vi "AlliGator Special Graph Menu Actions.vi"(8 "Error In":errorcluster, 9 "Help?":bool, 10 "Animated Busy Icon":bool, 11 "XY Graph Event":T1) -> (0 "Error Out":errorcluster, 1 "Message":string, 3 "AlliGator Actions":T3[](array[typedef]))   [LabVIEW 2021, in "AlliGator Graphs.lvlib"]
doc: "Additional graph menu items developped for AlliGator."
uses:
  AlliGator Graphs.lvlib
  AlliGator Q Element.ctl
  AlliGator Q Event.ctl
  Graphs/XY Graph/XY Graph Event.ctl
  <vilib>/Utility/miscctls.llb/LVPoint32TypeDef.ctl
  Graphs/XY Graph/XY Graph Selected Plot Info.ctl
  Graphs/XY Graph/XY Graph Refnum.ctl
  AlliGator Decay Graph Process Plot Target.ctl
  Graphs/XY Graph/XY Graph Selected Plot Info+Flag.ctl
  AlliGator Variables List.ctl
  Graphs/XY Graph/XY Graph Add-Ons.lvlib
  AlliGator Action Engine.lvlib
  AlliGator Python Plugins.lvlib
  AlliGator Decay Processing.lvlib
  AlliGator Decay Analysis.lvlib
  AlliGator Globals, Variables & Constants.lvlib
panel:
  # "see the AlliGator License on the block diagram (Ctrl+E or Window:Show Block Diagram)"
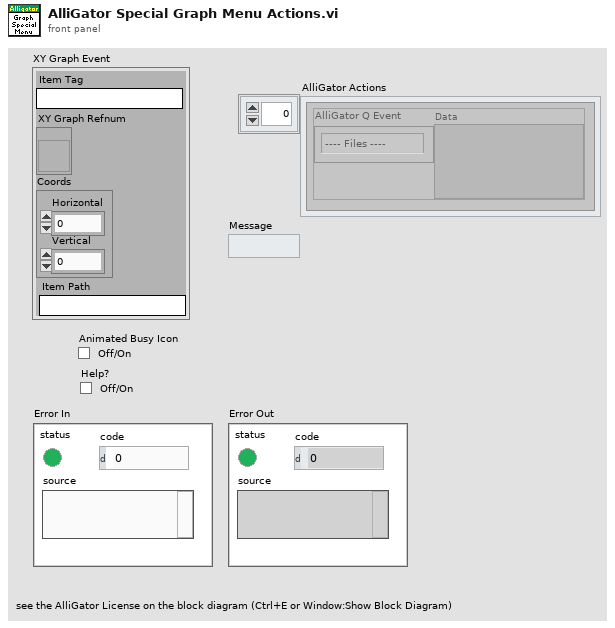
[diagram p1: front panel]
types:
  T1 = typedef "XY Graph Add-Ons.lvlib/XY Graph Event.ctl" = cluster{"Item Tag":string, "XY Graph Refnum":refnum<vi>, "Coords":T2, "Item Path":string}
  T2 = typedef "LVPoint32TypeDef.ctl" = cluster{"Horizontal":i32, "Vertical":i32}
  T3 = typedef "AlliGator Action Engine.lvlib/AlliGator Q Element.ctl" = cluster{"AlliGator Q Event":T4, "Data":variant}
  T4 = typedef "AlliGator Action Engine.lvlib/AlliGator Q Event.ctl" = enum16{"---- Files ----", "Files:Set Batch Export Files To Save", "Files:Set Dataset Loading & Pre-processing Options", "Files:Check #Frames in Dataset", "Files:Increment Frame Index", "Files:Open Mask Image", "Files:Open White Light Image", "Files:Open Single Dataset", "Files:New Folder of Folders Selected", "Files:Load File (all Types)_Scriptable", "Files:Move Flattened Series to Folders Series", "Files:Select Folder", "Files:Load FLI Dataset", "Files:Load Swiss SPAD 1 Dataset", "Files:Load Swiss SPAD 2 Dataset", "Files:Load .sdt FLI Dataset", "Files:Load .ptu FLI Dataset", "Files:Load .bin FLI Dataset", "Files:Load Single Gate Image Folder", "Files:Load I/m/phi Dataset (deprecated)", "Files:Load Single Image", "Files:Subtract Background File", "Files:Export FLI Dataset", "Files:Load HDF5 FLI Dataset", "Files:Set Destination File Path", "Files:Save Mask Image", "Files:Batch Conversion", "Files:New Folder Selected", "Files:Close FLI Dataset", "Files:Close FLI Dataset Series", "Files:Close White Light Image", "Files:Close Mask Image", "---- FLI Dataset ----", "FLI Dataset:Channel Arithmetic", "FLI Dataset:Export Average Lifetime Map as ASCII", "FLI Dataset:Export User-Defined Quantity Map as ASCII", "FLI Dataset:Python Function FLI Dataset Event", "FLI Dataset:ROI Analysis", "FLI Dataset:Tilted Logistic Square Gated IRF Characteristics Map", "FLI Dataset:Logistic Square Gated IRF Characteristics Map", "FLI Dataset:Square Gated IRF Characteristics Map", "FLI Dataset:Multi-ROI Single-Pixel Phasor Analysis", "FLI Dataset:Multi-ROI Single-Pixel NLSF Analysis", "FLI Dataset:All ROIs IRF Extraction", "FLI Dataset:All ROIs Decay Fit Non-Interactive (Fast + Individual IRF)", "FLI Dataset:All ROIs Phasor Analysis", "FLI Dataset:All ROIs Decay Fit", "FLI Dataset:Fluorescence Decay Statistics", "FLI Dataset:Update Decay Statistics Graph", "FLI Dataset:Get Decay from ROI", "FLI Dataset:All ROIs Average Lifetimes", "---- FLI Dataset Series ----", "FLI Dataset Series:Sum All Datasets in Series", "FLI Dataset Series:Add Dataset to Accumulated Dataset", "FLI Dataset Series:Display Accumulated Dataset", "FLI Dataset Series:Clear Dataset Series Sum", "FLI Dataset Series:Time-Series Analysis (NLSF)", "FLI Dataset Series:Time-Series Analysis (Phasor)", "---- Image ----", "Image:Update Image Profile Plots", "Image:Image Histogram Cursor Move", "Image:Image Histogram", "Image:Image Contrast", "Image:Set Image Histogram Cursor Move Flag", "Image:Clear Image Overlay", "Image:Use ROI as Search Area", "Image:Set ROI Diameter", "Image:Save Image Data as TIFF", "Image:Save Displayed Image with Overlay", "Image:Save Image Overlay Only", "Image:Save Image as Hot Pixel Mask", "Image:Change Source Image Color Palette", "Image:Copy Image to Clipboard", "Image:Source Image ROI Selection", "Image:Delete All ROIs", "Image:Delete All Unselected ROIs", "Image:Delete ROI", "Image:Merge All ROIs", "Image:Store ROI", "Image:Source Image ROI Storage", "Image:Export ROI Description to Notebook", "Image:Save ROI", "Image:Load ROI", "Image:Paste ROI Definition", "Image:Clear ROI", "Image:Identify ROIs in Mask Image", "Image:Create Complementary ROI", "Image:Create Contour ROI", "Image:Create ROI(s) from Pixels with Peak above Min_Scriptable", "Image:Create ROI(s) from Pixels with Intensity above Min_Scriptable", "Image:Compute ROI Statistics", "Image:Delete ROI(s) based on ROI Statistics", "Image:Create ROI Grid", "Image:ROI to Individual Pixel ROIs", "Image:Python Function Source Image Event", "Image:Show Phasor Calibration Map ROI Centers", "Image:Convert ROI to Mask Image", "Image:Mouse Move", "Image:Mouse Up", "Image:Set Source Image Mouse Move Flag", "Image:Add Scale Bar Overlay", "Image:Delete Existing ROIs Option", "---- Decay ----", "Decay:Clear IRF/Reference Plot", "Decay:Clear Local IRFs", "Decay:Add Decay to Graph", "Decay:Smoothen Plot", "Decay:Smoothen Plot Tail", "Decay:Average Selected Plots", "Decay:Extract IRF", "Decay:Optimal IRF Extraction", "Decay:Threshold IRF", "Decay:Fit to Model IRF", "Decay:Fit IRF to Square Gate", "Decay:Fit IRF to Logistic Square Gate", "Decay:Fit IRF to Tilted Logistic Square Gate", "Decay:Create Bounding Cursors Set", "Decay:Export Bounding Cursors Definition to Notebook", "Decay:Denoise Plot", "Decay:Compute Cumulative Function", "Decay:Use as Reference Decay", "Decay:Show Reference Decay/IRF", "Decay:Extrapolate Decay", "Decay:Create Head & Tail Bounding Cursors", "Decay:Store Cursor-defined Head & Tail Fractions", "Decay:Rebin Plot", "Decay:1-Normalize Decay", "Decay:[0-1]-Normalize Plot", "Decay:Straighten Decay", "Decay:Shift Decay", "Decay:Fold Decay", "Decay:Fit Decay", "Decay:Global Fit of Selected Decays", "Decay:Post Global Fit Script", "Decay:Add Global Fit Parameters to Graph", "Decay:Add Decay Parameter(s) to Plot (Graph)", "Decay:Export Decay to Phasor Graph", "Decay:Plot Decay Shifts", "Decay:Compute Average Lifetime", "Decay:Plot Convolution", "Decay:Graph Tip Strip Update", "---- Decay Statistics ----", "Decay Statistics:Tip Strip Update", "---- Intensity Time Trace ----", "Intensity Time Trace:Use File Timestamp", "Intensity Time Trace:Load Intensity Corrections File", "Intensity Time Trace:Clear Intensity Corrections File", "Intensity Time Trace:Tip Strip Update", "---- Phasor Plot ----", "Phasor Plot:Build Phasor Plot", "Phasor Plot:Change Phasor Plot Color Palette", "Phasor Plot:Adjust Phasor Plot Display Range", "Phasor Plot:Highlight Image ROI in Phasor Plot", "Phasor Plot:Save Phasor Plot Image with Overlay", "Phasor Plot:Export Complex Phasor Map", "Phasor Plot:Export Phasor Ratio Map", "Phasor Plot:Export Average Lifetime Map", "Phasor Plot:Compute Phase Lifetime Histogram", "Phasor Plot:Compute Phasor Ratio Histogram", "Phasor Plot:Compute Phase Lifetime vs Intensity Scatter Plot", "Phasor Plot:Weber 2-Component Decomposition", "Phasor Plot:Update Phasor Color Map Vertices", "Phasor Plot:Clear Phasor Overlay", "Phasor Plot:Use Segment Extremities as References", "Phasor Plot:Use UC/Segment Intersections as References", "Phasor Plot:Use UC/Principal Axis Intersections as References", "Phasor Plot:Use UC/Linear Fit Intersections as References", "Phasor Plot:Update Phasor Plot Reference", "Phasor Plot:Show Local Phasor Info in Phasor Plot", "Phasor Plot:Update Phasor Plot State", "Phasor Plot:Phasor Plot ROI Storage", "Phasor Plot:Phasor Plot ROI Selection", "Phasor Plot:Python Function Phasor Plot Event", "Phasor Plot:Overlay Phasor ROI, Ratio or Map in Source Image", "Phasor Plot:Phasor at Image Pixel", "Phasor Plot:Mouse Move", "Phasor Plot:Mouse Up", "Phasor Plot:Display Range Mouse Move", "Phasor Plot:Set Mouse Move Flag", "---- Phasor Graph ----", "Phasor Graph:Calibrated Phasor Map Series", "Phasor Graph:Whole Image Phasor Scatter Plot (Todo)", "Phasor Graph:Get Phasor Value", "Phasor Graph:Create New Phasor Plot Dialog", "Phasor Graph:Update Last Phasor Value", "Phasor Graph:Update Phasor (m, phi)", "Phasor Graph:Remove Single Phasor from Plot", "Phasor Graph:Add Single Phasor to Plot", "Phasor Graph:Remove Phasor Plot", "Phasor Graph:Remove Selected Phasor Plots", "Phasor Graph:Clear Phasor Data", "Phasor Graph:Clear Phasor Graph", "Phasor Graph:Cursor Move", "Phasor Graph:Draw Cursor Connecting Line", "Phasor Graph:Clear Cursor Connecting Line", "Phasor Graph:Find UC Intersection", "Phasor Graph:Use UC/Cursor-Defined Line Intersections", "Phasor Graph:Use Selected Plots Fitted Line/UC Intersections", "Phasor Graph:Use Selected Plots Principal Axis/UC Intersections", "Phasor Graph:Show Single Phasor", "Phasor Graph:Save Single Phasor Plot", "Phasor Graph:Save All Phasor Plots", "Phasor Graph:Load Phasor Plot(s)", "Phasor Graph:Phasor Multiplication", "Phasor Graph:Compute Average Phasor", "Phasor Graph:Compute Multiple Average Phasors (Selected Plots)", "Phasor Graph:Export Single Phasor Plot Phase Lifetimes", "Phasor Graph:Phase Lifetime Trajectory", "Phasor Graph:Phase Lifetime vs Intensity Scatter Plot (deprecated)", "Phasor Graph:Parameter 2 vs Parameter 1 Scatter Plot", "Phasor Graph:Use Cursor n Location", "Phasor Graph:Set Reference n to Current Phase Lifetime Value", "Phasor Graph:Set Reference n to Lifetime Value", "Phasor Graph:Set Cursor n Location", "Phasor Graph:Save Phasor Graph Image", "Phasor Graph:Update SEPL Plot", "Phasor Graph:Export Single Phasor Plot Data", "Phasor Graph:Export Selected Phasor Plots Data", "Phasor Graph:Python Function Phasor Graph Event", "Phasor Graph:Tip Strip Update", "---- Calibration ----", "Calibration:Set Calibration Type", "Calibration:Load/Save Phasor Calibration", "Calibration:Load/Save Phasor Calibration Series", "Calibration:Load/Save Phasor Calibration Map", "Calibration:Use as Calibration", "Calibration:Compute Optimal Calibration from Phasor References", "Calibration:Clear Phasor Calibration", "Calibration:Use as Calibration Series", "Calibration:Use as Calibration Map", "Calibration:Clear Calibration Series", "Calibration:Clear Calibration Map", "Calibration:Apply Phasor Calibration", "Calibration:Update Single Plot Calibration", "Calibration:Update Multiple Plots Calibration", "Calibration:Clear Single Plot Calibration", "Calibration:Clear All Plots Calibrations", "Calibration:Clear Plot(s) Calibration(s)?", "Calibration:Phasor Calibration Maps (# Gates Series)", "---- Phasor Ratio ----", "Phasor Ratio:Clear Reference n", "Phasor Ratio:Toggle Selected Plot(s)  Lock to Reference 1", "Phasor Ratio:Use as Reference n", "Phasor Ratio:Send Reference n to Notebook", "Phasor Ratio:Toggle Selected Plot(s)  Lock to Reference 2", "Phasor Ratio:Compute Phasor Ratio at Mouse Location", "Phasor Ratio:Compute Phasor Plot's Average Phasor Ratio", "Phasor Ratio:Compute Time-Series Phasor Ratios", "Phasor Ratio:Fit Line to Phasor Ratio Plot", "Phasor Ratio:Save References", "Phasor Ratio:Load References", "Phasor Ratio:Update Phasor Reference 1", "Phasor Ratio:Update Phasor Reference 2", "Phasor Ratio:Move Cursor n to Reference n", "Phasor Ratio:Use as Phasor Reference 1 Lifetime", "Phasor Ratio:Use as Phasor Reference 2 Lifetime", "Phasor Ratio:Export Phasor Ratio Map as ASCII", "Phasor Ratio:Tip Strip Update", "---- Lifetime & Other Parameters Graph ----", "Lifetime:Tip Strip Update", "---- Decay Fit Parameter Map ----", "Decay Fit Parameter Map:Export ROI NLSF Data as ASCII", "Decay Fit Parameter Map:Set Decay Fit  Parameter Map Selection", "Decay Fit Parameter Map:Build Decay Fit Parameter Map", "Decay Fit Parameter Map:Change Decay Fit Parameter Map Color Palette", "Decay Fit Parameter Map:Export Decay Fit Parameter Map Data as ASCII", "Decay Fit Parameter Map:Export All Decay Fit Parameter Maps Data as ASCII", "Decay Fit Parameter Map:Send Map Data to Lifetime Graph", "Decay Fit Parameter Map:Save Decay Fit Parameter Map Image", "Decay Fit Parameter Map:Save-Load IRFs & Fit Data", "Decay Fit Parameter Map:Update Local Decay Plots", "Decay Fit Parameter Map:Python Function Decay Fit Parameters Map Event", "Decay Fit Parameter Map:Overlay Decay Fit Parameter Map in Source Image", "Decay Fit Parameter Map:Plot Map Data vs Intensity", "Decay Fit Parameter Map:Mouse Up", "Decay Fit Parameter Map:Display Range Mouse Move", "---- Generic Graph ----", "Generic Graph:Generic XY Graph Event", "Generic Graph:Python Function XY Graph Event", "Generic Graph:New Plot", "Generic Graph:Save Plot", "Generic Graph:XY Plot Histogram", "Generic Graph:Set XY Graph Plot Name", "Generic Graph:Set Last Cursor Style", "Generic Graph:Tip Strip Update", "---- GUI ----", "GUI:Start Script", "GUI:Type of Displayed Image Changed", "GUI:Gate Image Slide Changed", "GUI:Show Busy Icon", "GUI:Show Busy Icon & Abort Button", "GUI:Hide Busy Icon", "GUI:Hide Busy Icon & Abort Button", "GUI:Abort", "GUI:End Script", "GUI:Start Timing", "GUI:End Timing", "GUI:Set State Indicator", "GUI:Send Parameters JSON Strings to Clipboard", "GUI:Set Gate Step", "GUI:Idle", "GUI:Initialization", "GUI:Quit", "GUI:Increment Dataset Index", "GUI:Set Dataset Index to -1", "GUI:Time Series Slider Moved", "GUI:Time Series Slider Changed", "GUI:Toggle Playback or Loop", "GUI:Playback Script", "GUI:Set Phasor Frequency", "GUI:Open Window", "DEBUG"}
  T5 = typedef "XY Graph Add-Ons.lvlib/XY Graph Selected Plot Info.ctl" = cluster{"Multiplot XY Graph":T6, "Mouse Coordinates":T2, "Plot Index":i32}
  T6 = typedef "XY Graph Add-Ons.lvlib/XY Graph Refnum.ctl" = refnum<vi>
  T7 = typedef "AlliGator Decay Analysis.lvlib/AlliGator Decay Graph Process Plot Target.ctl" = enum16{"Single Plot", "Selected Plots", "All Plots"}
  T8 = typedef "XY Graph Add-Ons.lvlib/XY Graph Selected Plot Info+Flag.ctl" = cluster{"Multiplot XY Graph":T6, "Mouse Coordinates":T2, "Plot Index":i32, "Flag":bool}
  T9 = typedef "AlliGator Globals, Variables & Constants.lvlib/AlliGator Variables List.ctl" = enum16{"---- GUI ----", "Initialization Status", "State Indicators Refnum", "Original AlliGator Menu Items", "Current Action Loop State", "Script in progress", "Playback", "Loop Playback", "Search ROI Used", "Search ROI", "Decay Graph Max Legend Size", "Intensity Graph Max Legend Size", "Decay Statistics Graph Max Legend Size", "Phasor Graph Max Legend Size", "Phasor Ratio Graph Max Legend Size", "Lifetime Graph Max Legend Size", "---- Files ----", "Export Dataset Frames as Individual Files", "Show Batch Export Help Balloons", "Frames in Dataset", "ptu File Frame Start Indices", "Current Frame in Dataset", "Current Frame Timestamp", "------ Python Plugins ------", "Python Plugins Information", "Python Session", "Valid Python Session?", "---- Source Image ----", "Dataset Loaded", "Dataset Metadata", "Dataset Channel", "Dataset Data Description", "Background Dataset Metadata", "Background Dataset Channel", "Background Dataset Data Description", "Background File Subtraction", "Background File Path", "Background File Pile-up Correction", "Background File Pixel Well Capacity", "Background File Scaling Factor", "Source Image ROIs", "Current Source Image ROI", "Source Image ROI Event Refnum", "X_Source Image Display Range", "X_Source Image Palette Information", "Source Image Palette List", "Source Image Scale", "Current Dataset Load Settings", "Source Image:ROI Overlay Color", "---- Image Profile Window ----", "Image Profile:Overlay ROI in Source Image", "Image Profile Window Event Refnum", "Image Profile:IntensityType", "Image Profile:Intensity Average Type", "Image Profile:Intensity-weighted SDV", "Image Profile:Box Profile Type", "Image Profile Window Open", "Image Profile:Plotted Fit Parameter", "X_Type of Displayed Image", "X_Time Gate Slider", "Dataset Path", "Source Image Overlay to Erase", "Is Displayed Image Accumulated", "White Light Image Modified", "Mask Image Modified", "Macrotime Gate Separation", "------ Phasor Graph -------", "Phasor Graph:Show Line", "---- Phasor Plot ---", "Phasor Plot Parameters Changed", "FLI Dataset Modified since last Phasor Plot Calculation", "Phasor Harmonics Data", "Selected Phasor Harmonics", "Phasor Harmonic Manager Event Refnum", "Phasor Plot ROIs", "Current Phasor Plot ROI", "Phasor Plot ROI Event Refnum", "Phasor Plot Image Reference Points", "Phasor Plot Computed", "Phasor Plot Palette Information", "Phasor Plot Palette List", "Phasor Ratio Palette Information", "Phasor Ratio Palette List", "Phasor Image Scale", "Phasor Plot Image Overlay to Erase", "Phasor Plot Image Elements to Update", "Current Phasor Plot Calculation Parameters", "Current Phasor Calibration Options", "Reset Cumulated Phasor Plot", "Phasor Ratio Reference 1", "Phasor Ratio Lifetime Reference 1", "Phasor Ratio Reference 1 Frequency", "Phasor Ratio Reference 2", "Phasor Ratio Lifetime Reference 2", "Phasor Ratio Reference 2 Frequency", "---- Decay Analysis ----", "Number of Selected Decays to Fit", "LS Fit Results", "LAR Fit Results", "BS Fit Results", "Last Decay Max - Min", "Best Fit Parameters", "Best Fit Parameter Names", "Actual Size X", "Actual Size Y", "Binning X", "Binning Y", "Actual # Gates", "Dataset Number", "Gates to...", "Gates Skipped", "Gates to keep", "Gate Step", "Gate Separation", "Reversed Gates", "Pile-up Correction", "Pixel Well Capacity", "Background Subtracted", "Background Subtraction Method", "Background Definition Range", "Background File (deprecated)", "Number of Dataset Accumulated", "Array of Accumulated Dataset Paths", "Do Averaged Datasets", "Destination File Path", "Process Plot Target", "Use 1/D as Phasor Frequency", "---- Decay Fit Parameter Map -----", "Decay Fit Parameter Map Palette Information", "Decay Fit Parameter Map Palette List", "Local Decay Graph Window Event Refnum", "------- Local Decay Window ---------", "Use normalized IRF for convolution", "----- Miscellaneous ----", "Skippable Dialog Windows Status"}
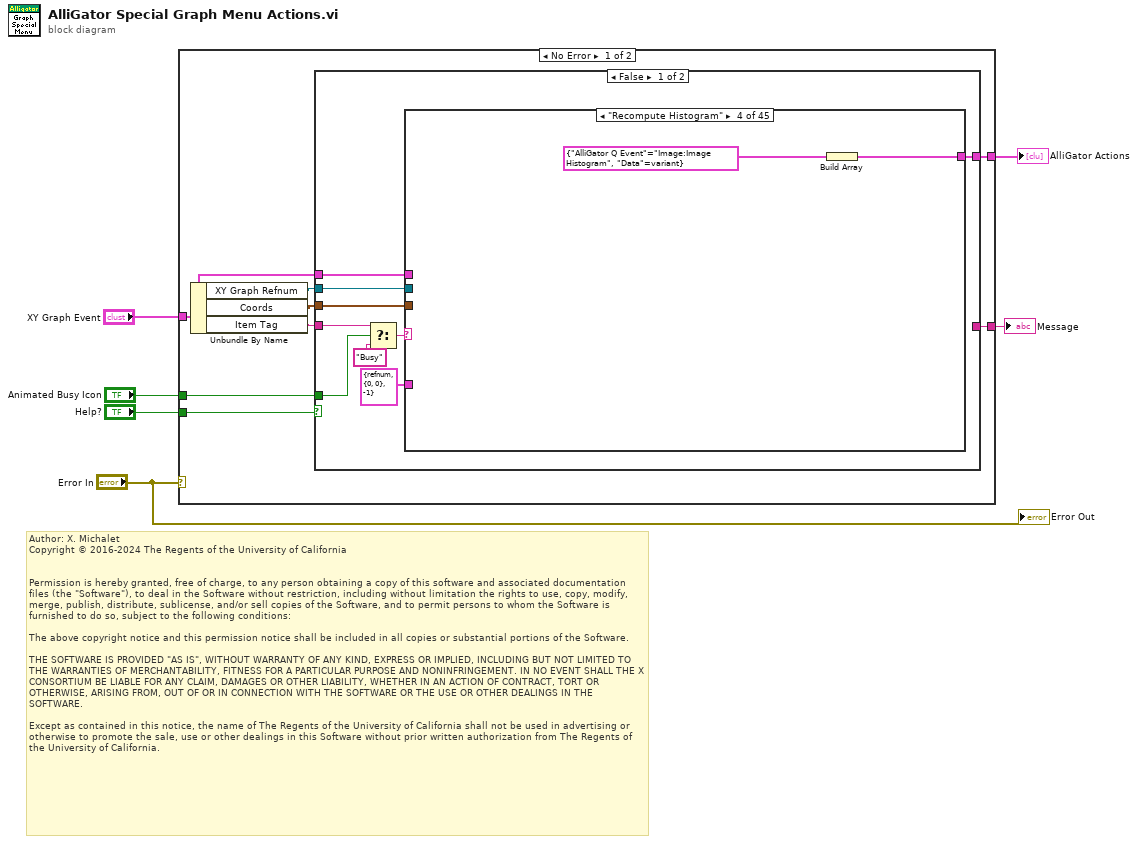
[diagram p0: block diagram]
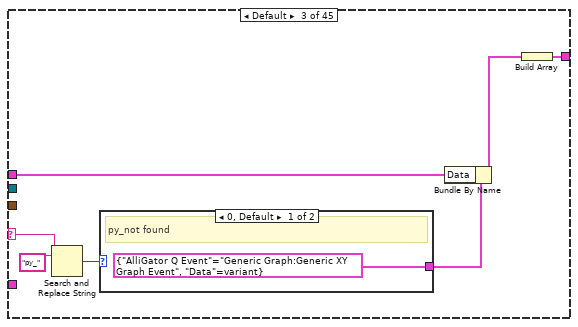
[diagram p4: hidden frame]
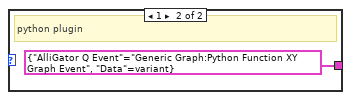
[diagram p5: hidden frame]
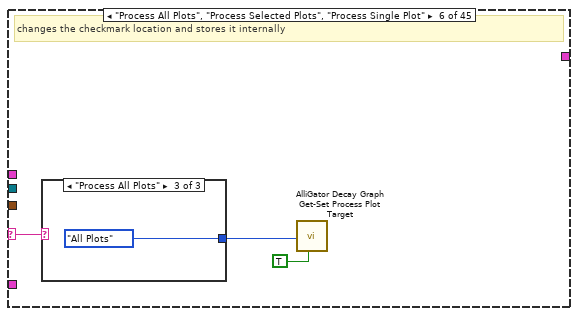
[diagram p7: hidden frame]
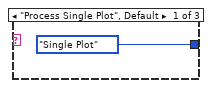
[diagram p8: hidden frame]
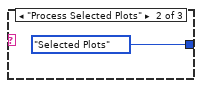
[diagram p9: hidden frame]
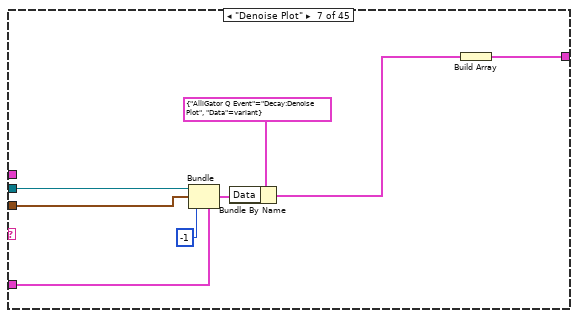
[diagram p10: hidden frame]
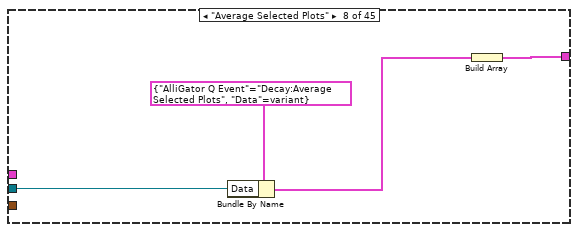
[diagram p11: hidden frame]
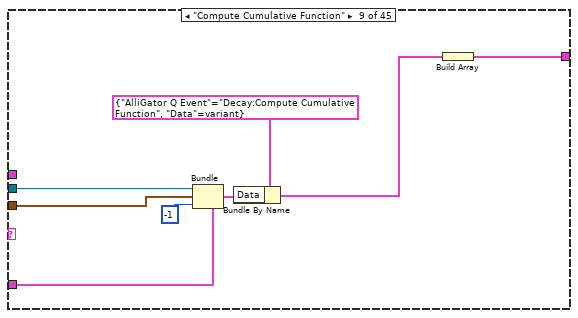
[diagram p12: hidden frame]
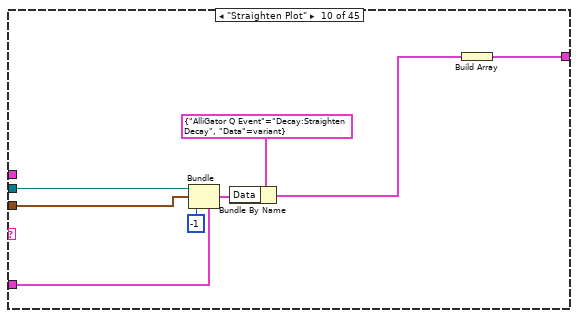
[diagram p13: hidden frame]
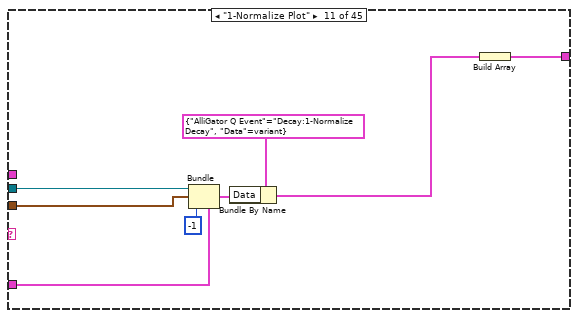
[diagram p14: hidden frame]
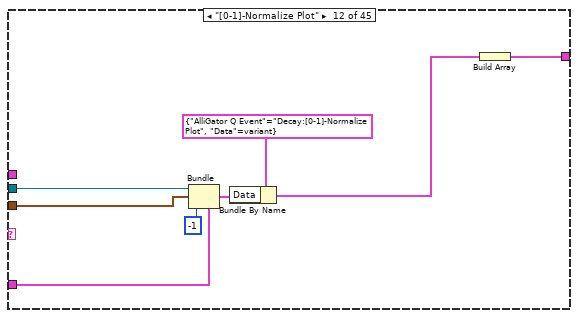
[diagram p15: hidden frame]
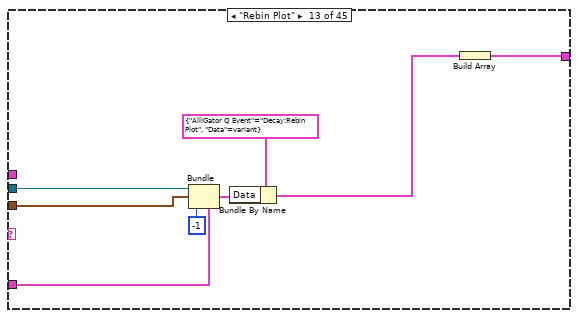
[diagram p16: hidden frame]
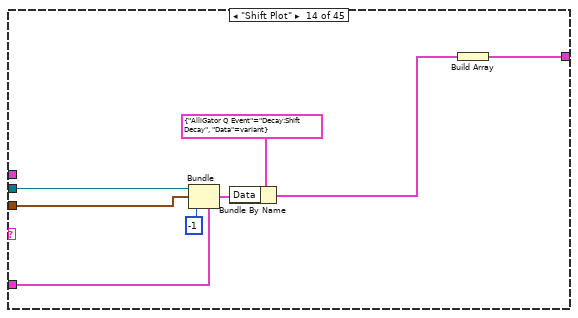
[diagram p17: hidden frame]
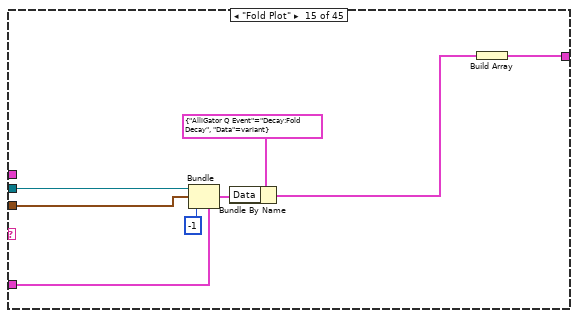
[diagram p18: hidden frame]
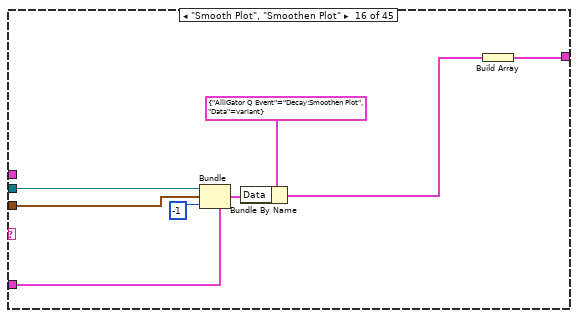
[diagram p19: hidden frame]
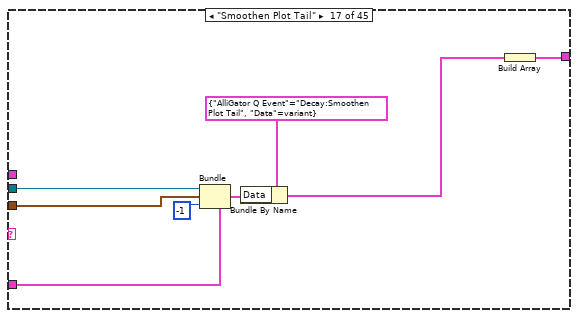
[diagram p20: hidden frame]
diagram:
  # "Author: X. Michalet\nCopyright © 2016-2024 The Regents of the University of California\n \n\nPermission is hereby granted, free of charge, to any person obtaining a copy of this software and associated documentation files (the \"Software\"), to deal in the Software without restriction, including without limitation the rights to use, copy, modify, merge, publish, distribute, sublicense, and/or sell copies of the Software, and to permit persons to whom the Software is furnished to do so, subject to the following conditions:\n\nThe above copyright notice and this permission notice shall be included in all copies or substantial portions of the Software.\n\nTHE SOFTWARE IS PROVIDED \"AS IS\", WITHOUT WARRANTY OF ANY KIND, EXPRESS OR IMPLIED, INCLUDING BUT NOT LIMITED TO THE WARRANTIES OF MERCHANTABILITY, FITNESS FOR A PARTICULAR PURPOSE AND NONINFRINGEMENT. IN NO EVENT SHALL THE X CONSORTIUM BE LIABLE FOR ANY CLAIM, DAMAGES OR OTHER LIABILITY, WHETHER IN AN ACTION OF CONTRACT, TORT OR OTHERWISE, ARISING FROM, OUT OF OR IN CONNECTION WITH THE SOFTWARE OR THE USE OR OTHER DEALINGS IN THE SOFTWARE.\n\nExcept as contained in this notice, the name of The Regents of the University of California shall not be used in advertising or otherwise to promote the sale, use or other dealings in this Software without prior written authorization from The Regents of the University of California."
  n1 = case shown="No Error" "Error In" {
    tunnel: [w14 _] -> w6
    tunnel: "Help?" -> [w13 _]
    tunnel: "Animated Busy Icon" -> [w12 _]
    tunnel: "XY Graph Event" -> [w8 _]
    tunnel: [w7 _] -> w1
    frame No Error {
      n2 = Unbundle By Name(w8) -> ("XY Graph Refnum"=w11:refnum<vi>, "Coords"=w10:T2, "Item Tag"=w9:string)
      n3 = case shown="False" w13 {
        tunnel: w12 -> [w23 _]
        tunnel: w9 -> [w21 w279]
        tunnel: w11 -> [w20 w281]
        tunnel: w10 -> [w19 _]
        tunnel: [w17 _] -> w14
        tunnel: w8 -> [w15 _]
        tunnel: [_ w278] -> w7
        frame False {
          n4 = Select(t=w21, s=w23, f="Busy" ("t")) -> (s? t:f=w22:string)
          n5 = case shown="\"Recompute Histogram\"" w22 {
            selector: w22 -> [_ _ w24 _ _ w37 _ _ _ _ _ _ _ _ _ _ _ _ _ _ _ _ _ _ _ _ _ _ _ _ _ _ _ _ _ _ _ _ _ _ _ _ _ _ _]
            tunnel: w20 -> [_ _ _ _ _ _ w46 w50 w58 w66 w74 w82 w90 w98 w106 w114 w122 w130 _ w140 w148 _ w156 _ w164 w172 w180 w188 w196 w202 w216 w224 _ _ _ w236 _ _ _ _ w251 _ _ w261 w272]
            tunnel: w19 -> [_ _ _ _ _ _ w44 _ w56 w64 w72 w80 w88 w96 w104 w112 w120 w128 _ w139 w147 _ w155 _ w162 w170 w178 w186 w194 w201 w214 w222 _ _ _ w234 _ _ _ _ w249 _ _ w260 w271]
            tunnel: T5 {"Multiplot XY Graph"=refnum, "Mouse Coordinates"={"Horizontal"=0, "Vertical"=0}, "Plot Index"=-1} ("Selected Plot Info") -> [_ _ _ _ _ _ w42 _ w54 w62 w70 w78 w86 w94 w102 w110 w118 w126 _ w135 w143 _ w151 _ w160 w168 w176 w184 w192 w200 w212 w220 _ _ _ w232 _ _ _ _ _ _ _ w262 w273]
            tunnel: [_ _ w26 w33 _ _ w41 w49 w53 w61 w69 w77 w85 w93 w101 w109 w117 w125 w133 w136 w144 _ w152 _ w159 w167 w175 w183 w191 w199 w211 w219 w227 w229 _ w231 w239 w242 w244 _ w245 w254 _ w259 w270] -> w17
            tunnel: w15 -> [_ _ w25 _ _ _ _ _ _ _ _ _ _ _ _ _ _ _ _ _ _ _ _ _ _ _ _ _ _ _ _ _ _ _ _ _ _ _ _ _ _ _ _ _ _]
            frame "-" {
            }
            frame "Busy" {
            }
            frame Default {
              n6 = Search and Replace String(input string=w24, search string="py_") -> (number of replacements=w27:i32)  [unwired: 6 in, 3 out]
              n7 = case shown="0, Default" w27 {
                tunnel: [T3 {"AlliGator Q Event"=enum."Generic Graph:Generic XY Graph Event", "Data"=variant} ("element") T3 {"AlliGator Q Event"=enum."Generic Graph:Python Function XY Graph Event", "Data"=variant} ("element")] -> w29
                frame 0, Default {
                  # "py_not found"
                }
                frame 1 {
                  # "python plugin"
                }
              }
              n8 = Bundle By Name(cluster=w29, "Data"=w25) -> (w28:T3)
              n9 = Build Array(w28) -> (w26:T3[])
            }
            frame "Recompute Histogram" {
              n10 = Build Array(T3 {"AlliGator Q Event"=enum."Image:Image Histogram", "Data"=variant} ("element")) -> (w33:T3[])
            }
            frame "---------------------" {
            }
            frame "Process All Plots", "Process Selected Plots", "Process Single Plot" {
              # "changes the checkmark location and stores it internally"
              n11 = case shown="\"Process All Plots\"" w37 {
                tunnel: [AlliGator_Decay_Graph_Process_Plot_Target."Single Plot" ("Process Plot Target") AlliGator_Decay_Graph_Process_Plot_Target."Selected Plots" ("Process Plot Target") AlliGator_Decay_Graph_Process_Plot_Target."All Plots" ("Process Plot Target")] -> w36
                frame "Process Single Plot", Default {
                }
                frame "Process Selected Plots" {
                }
                frame "Process All Plots" {
                }
              }
              n12 = call "AlliGator Decay Graph Get-Set Process Plot Target.vi"("Get (F)/Set"=TRUE, "Plot(s) to Process in"=w36) -> ()  [unwired: 7 in, 3 out]
            }
            frame "Denoise Plot" {
              n13 = Bundle(cluster=w42, "Multiplot XY Graph"=w46, "Mouse Coordinates"=w44, "Plot Index"=-1) -> (w45:T5)
              n14 = Bundle By Name(cluster=T3 {"AlliGator Q Event"=enum."Decay:Denoise Plot", "Data"=variant} ("element"), "Data"=w45) -> (w47:T3)
              n15 = Build Array(w47) -> (w41:T3[])
            }
            frame "Average Selected Plots" {
              n16 = Bundle By Name(cluster=T3 {"AlliGator Q Event"=enum."Decay:Average Selected Plots", "Data"=variant} ("element"), "Data"=w50) -> (w51:T3)
              n17 = Build Array(w51) -> (w49:T3[])
            }
            frame "Compute Cumulative Function" {
              n18 = Bundle(cluster=w54, "Multiplot XY Graph"=w58, "Mouse Coordinates"=w56, "Plot Index"=-1) -> (w57:T5)
              n19 = Bundle By Name(cluster=T3 {"AlliGator Q Event"=enum."Decay:Compute Cumulative Function", "Data"=variant} ("element"), "Data"=w57) -> (w59:T3)
              n20 = Build Array(w59) -> (w53:T3[])
            }
            frame "Straighten Plot" {
              n21 = Bundle(cluster=w62, "Multiplot XY Graph"=w66, "Mouse Coordinates"=w64, "Plot Index"=-1) -> (w65:T5)
              n22 = Bundle By Name(cluster=T3 {"AlliGator Q Event"=enum."Decay:Straighten Decay", "Data"=variant} ("element"), "Data"=w65) -> (w67:T3)
              n23 = Build Array(w67) -> (w61:T3[])
            }
            frame "1-Normalize Plot" {
              n24 = Bundle(cluster=w70, "Multiplot XY Graph"=w74, "Mouse Coordinates"=w72, "Plot Index"=-1) -> (w73:T5)
              n25 = Bundle By Name(cluster=T3 {"AlliGator Q Event"=enum."Decay:1-Normalize Decay", "Data"=variant} ("element"), "Data"=w73) -> (w75:T3)
              n26 = Build Array(w75) -> (w69:T3[])
            }
            frame "[0-1]-Normalize Plot" {
              n27 = Bundle(cluster=w78, "Multiplot XY Graph"=w82, "Mouse Coordinates"=w80, "Plot Index"=-1) -> (w81:T5)
              n28 = Bundle By Name(cluster=T3 {"AlliGator Q Event"=enum."Decay:[0-1]-Normalize Plot", "Data"=variant} ("element"), "Data"=w81) -> (w83:T3)
              n29 = Build Array(w83) -> (w77:T3[])
            }
            frame "Rebin Plot" {
              n30 = Bundle(cluster=w86, "Multiplot XY Graph"=w90, "Mouse Coordinates"=w88, "Plot Index"=-1) -> (w89:T5)
              n31 = Bundle By Name(cluster=T3 {"AlliGator Q Event"=enum."Decay:Rebin Plot", "Data"=variant} ("element"), "Data"=w89) -> (w91:T3)
              n32 = Build Array(w91) -> (w85:T3[])
            }
            frame "Shift Plot" {
              n33 = Bundle(cluster=w94, "Multiplot XY Graph"=w98, "Mouse Coordinates"=w96, "Plot Index"=-1) -> (w97:T5)
              n34 = Bundle By Name(cluster=T3 {"AlliGator Q Event"=enum."Decay:Shift Decay", "Data"=variant} ("element"), "Data"=w97) -> (w99:T3)
              n35 = Build Array(w99) -> (w93:T3[])
            }
            frame "Fold Plot" {
              n36 = Bundle(cluster=w102, "Multiplot XY Graph"=w106, "Mouse Coordinates"=w104, "Plot Index"=-1) -> (w105:T5)
              n37 = Bundle By Name(cluster=T3 {"AlliGator Q Event"=enum."Decay:Fold Decay", "Data"=variant} ("element"), "Data"=w105) -> (w107:T3)
              n38 = Build Array(w107) -> (w101:T3[])
            }
            frame "Smooth Plot", "Smoothen Plot" {
              n39 = Bundle(cluster=w110, "Multiplot XY Graph"=w114, "Mouse Coordinates"=w112, "Plot Index"=-1) -> (w113:T5)
              n40 = Bundle By Name(cluster=T3 {"AlliGator Q Event"=enum."Decay:Smoothen Plot", "Data"=variant} ("element"), "Data"=w113) -> (w115:T3)
              n41 = Build Array(w115) -> (w109:T3[])
            }
            frame "Smoothen Plot Tail" {
              n42 = Bundle(cluster=w118, "Multiplot XY Graph"=w122, "Mouse Coordinates"=w120, "Plot Index"=-1) -> (w121:T5)
              n43 = Bundle By Name(cluster=T3 {"AlliGator Q Event"=enum."Decay:Smoothen Plot Tail", "Data"=variant} ("element"), "Data"=w121) -> (w123:T3)
              n44 = Build Array(w123) -> (w117:T3[])
            }
            frame "Extrapolate Plot" {
              n45 = Bundle(cluster=w126, "Multiplot XY Graph"=w130, "Mouse Coordinates"=w128, "Plot Index"=-1) -> (w129:T5)
              n46 = Bundle By Name(cluster=T3 {"AlliGator Q Event"=enum."Decay:Extrapolate Decay", "Data"=variant} ("element"), "Data"=w129) -> (w131:T3)
              n47 = Build Array(w131) -> (w125:T3[])
            }
            frame "Create Head & Tail Bounding Cursors" {
              n48 = Build Array(T3 {"AlliGator Q Event"=enum."Decay:Create Head & Tail Bounding Cursors", "Data"=variant} ("element")) -> (w133:T3[])
            }
            frame "Store Cursor-defined Head & Tail Fractions" {
              n49 = Bundle(cluster=w135, "Multiplot XY Graph"=w140, "Mouse Coordinates"=w139, "Plot Index"=-1) -> (w142:T5)
              n50 = Bundle By Name(cluster=T3 {"AlliGator Q Event"=enum."Decay:Store Cursor-defined Head & Tail Fractions", "Data"=variant} ("element"), "Data"=w142) -> (w137:T3)
              n51 = Build Array(w137) -> (w136:T3[])
            }
            frame "Plot Convolution" {
              n52 = Bundle(cluster=w143, "Multiplot XY Graph"=w148, "Mouse Coordinates"=w147, "Plot Index"=-1) -> (w150:T5)
              n53 = Bundle By Name(cluster=T3 {"AlliGator Q Event"=enum."Decay:Plot Convolution", "Data"=variant} ("element"), "Data"=w150) -> (w145:T3)
              n54 = Build Array(w145) -> (w144:T3[])
            }
            frame "------------------" {
            }
            frame "Compute Average Lifetime" {
              n55 = Bundle(cluster=w151, "Multiplot XY Graph"=w156, "Mouse Coordinates"=w155, "Plot Index"=-1) -> (w158:T5)
              n56 = Bundle By Name(cluster=T3 {"AlliGator Q Event"=enum."Decay:Compute Average Lifetime", "Data"=variant} ("element"), "Data"=w158) -> (w153:T3)
              n57 = Build Array(w153) -> (w152:T3[])
            }
            frame "------- IRF -------" {
            }
            frame "Extract IRF by Deconvolution (Fixed Tau)" {
              n58 = Bundle(cluster=w160, "Multiplot XY Graph"=w164, "Mouse Coordinates"=w162, "Plot Index"=-1) -> (w163:T5)
              n59 = Bundle By Name(cluster=T3 {"AlliGator Q Event"=enum."Decay:Extract IRF", "Data"=variant} ("element"), "Data"=w163) -> (w165:T3)
              n60 = Build Array(w165) -> (w159:T3[])
            }
            frame "Compute Optimal Deconvolution IRF" {
              n61 = Bundle(cluster=w168, "Multiplot XY Graph"=w172, "Mouse Coordinates"=w170, "Plot Index"=-1) -> (w171:T5)
              n62 = Bundle By Name(cluster=T3 {"AlliGator Q Event"=enum."Decay:Optimal IRF Extraction", "Data"=variant} ("element"), "Data"=w171) -> (w173:T3)
              n63 = Build Array(w173) -> (w167:T3[])
            }
            frame "Fit IRF to Gaussian*Exponential Model" {
              n64 = Bundle(cluster=w176, "Multiplot XY Graph"=w180, "Mouse Coordinates"=w178, "Plot Index"=-1) -> (w179:T5)
              n65 = Bundle By Name(cluster=T3 {"AlliGator Q Event"=enum."Decay:Fit to Model IRF", "Data"=variant} ("element"), "Data"=w179) -> (w181:T3)
              n66 = Build Array(w181) -> (w175:T3[])
            }
            frame "Threshold IRF" {
              n67 = Bundle(cluster=w184, "Multiplot XY Graph"=w188, "Mouse Coordinates"=w186, "Plot Index"=-1) -> (w187:T5)
              n68 = Bundle By Name(cluster=T3 {"AlliGator Q Event"=enum."Decay:Threshold IRF", "Data"=variant} ("element"), "Data"=w187) -> (w189:T3)
              n69 = Build Array(w189) -> (w183:T3[])
            }
            frame "Fit IRF to Square Gate" {
              n70 = Bundle(cluster=w192, "Multiplot XY Graph"=w196, "Mouse Coordinates"=w194, "Plot Index"=-1) -> (w195:T5)
              n71 = Bundle By Name(cluster=T3 {"AlliGator Q Event"=enum."Decay:Fit IRF to Square Gate", "Data"=variant} ("element"), "Data"=w195) -> (w197:T3)
              n72 = Build Array(w197) -> (w191:T3[])
            }
            frame "Fit to Cubic Spline + Sine" {
              n73 = disable-structure shown="Disabled" {
                disable-tunnel: w202 -> [w208 _]
                disable-tunnel: w201 -> [w206 _]
                disable-tunnel: w200 -> [w204 _]
                disable-tunnel: [w203 _] -> w199
                frame Disabled {
                  n74 = Bundle(cluster=w204, "Multiplot XY Graph"=w208, "Mouse Coordinates"=w206, "Plot Index"=-1) -> (w207:T5)
                  n75 = Bundle By Name(cluster=T3 {"AlliGator Q Event"=enum."DEBUG", "Data"=variant} ("element"), "Data"=w207) -> (w209:T3)
                  n76 = Build Array(w209) -> (w203:T3[])
                }
                frame Enabled {
                }
              }
            }
            frame "Fit IRF to Logistic Square Gate" {
              n77 = Bundle(cluster=w212, "Multiplot XY Graph"=w216, "Mouse Coordinates"=w214, "Plot Index"=-1) -> (w215:T5)
              n78 = Bundle By Name(cluster=T3 {"AlliGator Q Event"=enum."Decay:Fit IRF to Logistic Square Gate", "Data"=variant} ("element"), "Data"=w215) -> (w217:T3)
              n79 = Build Array(w217) -> (w211:T3[])
            }
            frame "Fit IRF to Tilted Logistic Square Gate" {
              n80 = Bundle(cluster=w220, "Multiplot XY Graph"=w224, "Mouse Coordinates"=w222, "Plot Index"=-1) -> (w223:T5)
              n81 = Bundle By Name(cluster=T3 {"AlliGator Q Event"=enum."Decay:Fit IRF to Tilted Logistic Square Gate", "Data"=variant} ("element"), "Data"=w223) -> (w225:T3)
              n82 = Build Array(w225) -> (w219:T3[])
            }
            frame "Create Bounding Cursors Set" {
              n83 = Build Array(T3 {"AlliGator Q Event"=enum."Decay:Create Bounding Cursors Set", "Data"=variant} ("element")) -> (w227:T3[])
            }
            frame "Export Bounding Cursors Definition to Notebook" {
              n84 = Build Array(T3 {"AlliGator Q Event"=enum."Decay:Export Bounding Cursors Definition to Notebook", "Data"=variant} ("element")) -> (w229:T3[])
            }
            frame "--------------" {
            }
            frame "Use as Reference Plot" {
              w233 = -1  # User Interaction
              n85 = Bundle(cluster=w232, "Multiplot XY Graph"=w236, "Mouse Coordinates"=w234, "Plot Index"=w233) -> (w235:T5)
              n86 = Bundle By Name(cluster=T3 {"AlliGator Q Event"=enum."Decay:Use as Reference Decay", "Data"=variant} ("element"), "Data"=w235) -> (w237:T3)
              n87 = Build Array(w237) -> (w231:T3[])
            }
            frame "Show Reference Plot", "Show Reference Plot/IRF" {
              n88 = Build Array(T3 {"AlliGator Q Event"=enum."Decay:Show Reference Decay/IRF", "Data"=variant} ("element")) -> (w239:T3[])
            }
            frame "Clear IRF/Reference Plot" {
              n89 = Build Array(T3 {"AlliGator Q Event"=enum."Decay:Clear IRF/Reference Plot", "Data"=variant} ("element")) -> (w242:T3[])
            }
            frame "Clear Local IRFs" {
              n90 = Build Array(T3 {"AlliGator Q Event"=enum."Decay:Clear Local IRFs", "Data"=variant} ("element")) -> (w244:T3[])
            }
            frame "----------------" {
            }
            frame "Fit Plot" {
              w246 = TRUE  # Interactive
              w248 = -1  # User Interaction
              n91 = Bundle(cluster=T8 {"Multiplot XY Graph"=refnum, "Mouse Coordinates"={"Horizontal"=0, "Vertical"=0}, "Plot Index"=-1, "Flag"=FALSE} ("Selected Plot Info + Flag"), "Multiplot XY Graph"=w251, "Mouse Coordinates"=w249, "Plot Index"=w248, "Flag"=w246) -> (w250:T8)
              n92 = Bundle By Name(cluster=T3 {"AlliGator Q Event"=enum."Decay:Fit Decay", "Data"=variant} ("element"), "Data"=w250) -> (w252:T3)
              n93 = Build Array(w252) -> (w245:T3[])
            }
            frame "Global Fit of Selected Plots" {
              n94 = Build Array(T3 {"AlliGator Q Event"=enum."Decay:Global Fit of Selected Decays", "Data"=variant} ("element")) -> (w254:T3[])
            }
            frame "--------------------" {
            }
            frame "Using Current Phasor Frequency" {
              # "\"Export Plot's Phasor to Phasor Graph\""
              n95 = Bundle(cluster=w262, "Multiplot XY Graph"=w261, "Mouse Coordinates"=w260, "Plot Index"=-1) -> (w264:T5)
              n96 = Bundle By Name(cluster=T3 {"AlliGator Q Event"=enum."Decay:Export Decay to Phasor Graph", "Data"=variant} ("element"), "Data"=w264) -> (w265:T3)
              n97 = call "Alligator Variables Storage.vi"("Get(F)/Set"=TRUE, "AlliGator Variable"=AlliGator_Variables_List."Use 1/D as Phasor Frequency", "Data in"=FALSE ("Get(F)/Set")) -> ()  [unwired: 6 in, 3 out]
              n98 = Build Array(w265) -> (w259:T3[])
            }
            frame "Using f = 1/D" {
              # "\"Export Plot's Phasor to Phasor Graph\""
              n99 = Bundle(cluster=w273, "Multiplot XY Graph"=w272, "Mouse Coordinates"=w271, "Plot Index"=-1) -> (w275:T5)
              n100 = Bundle By Name(cluster=T3 {"AlliGator Q Event"=enum."Decay:Export Decay to Phasor Graph", "Data"=variant} ("element"), "Data"=w275) -> (w276:T3)
              n101 = call "Alligator Variables Storage.vi"("Get(F)/Set"=TRUE, "AlliGator Variable"=AlliGator_Variables_List."Use 1/D as Phasor Frequency", "Data in"=TRUE ("Get(F)/Set")) -> ()  [unwired: 6 in, 3 out]
              n102 = Build Array(w276) -> (w270:T3[])
            }
          }
        }
        frame True {
          # "Send Doc String of Python Plugin to Notebook"
          n103 = property class="XYGraph (strict)"(reference=w281) -> ("Label.Text"=w280:string)  [unwired: 1 in, 2 out]
          n104 = call "AlliGator Send Python Function Doc String to Notebook.vi"("Item Tag"=w279, "Target"=w280) -> ("Message"=w278:string)  [unwired: 8 in, 1 out]
        }
      }
    }
    frame Error {
    }
  }
  "AlliGator Actions" <- w6
  "Message" <- w1
  "Error Out" <- "Error In"
